vi "Write Execution time.vi"(10 "Method Start Time":timestamp, 11 "Method Result In":refnum<class "Method Result.lvclass">) -> (3 "Method Result Out":refnum<class "Method Result.lvclass">)   [LabVIEW 2020, in "Method Result.lvclass"]
uses:
  Method Result.lvclass
  Method Result.lvclass/Method Result.ctl
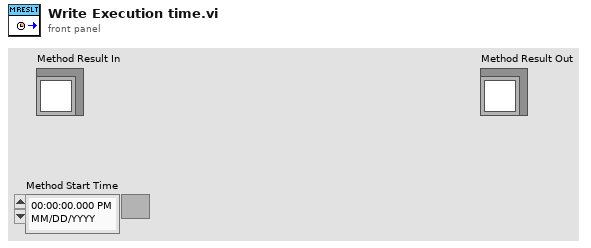
[diagram p1: front panel]
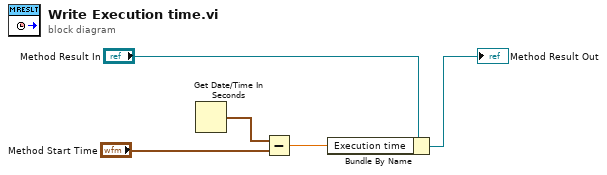
[diagram p0: block diagram]
diagram:
  n1 = Get Date/Time In Seconds() -> (seconds since 1Jan1904=w3:timestamp)
  n2 = Subtract(x=w3, y="Method Start Time") -> (x-y=w2:dbl)
  n3 = Bundle By Name(cluster="Method Result In", "Execution time"=w2) -> (→"Method Result Out":refnum<class "Method Result.lvclass">)
